vi "Thermometer Readout.vi"() -> ()   [LabVIEW 2023]
uses:
  <vilib>/Utility/file.llb/Read Delimited Spreadsheet (DBL).vi
  MQM Data Transfer All.vi
  Global Variables/Thermometers.vi
panel:
  out "Calibration confirmed":bool
  out "R_H Log Domain":dbl[](array[numeric])
  out "R_H coeffs":dbl[](array[numeric])
  out "Temperatures":cluster{"T_H":dbl, "T_C1":dbl, "T_C2":dbl}
  in  "Stop":bool
  in  "Delay (ms)":dbl=300.0
  in  "T_C2 Lockin":enum16{"LI1", "LI2", "LI3"}(ring)=enum."LI3"
  in  "I_therm":dbl
  in  "T_C1 Lockin":enum16{"LI1", "LI2", "LI3"}(ring)=enum."LI2"
  in  "T_H Lockin":enum16{"LI1", "LI2", "LI3"}(ring)
  out "R_C2 Log Domain":dbl[](array[numeric])
  out "R_C1 Log Domain":dbl[](array[numeric])
  out "R_C2 coeffs":dbl[](array[numeric])
  out "R_C1 coeffs":dbl[](array[numeric])
  in  "R_H domain file":path
  in  "R_C2 domain file":path
  in  "R_C1 domain file":path
  in  "R_C2 coeffs file":path
  in  "R_C1 coeffs file":path
  in  "R_H coeffs file":path
  in  "Confirm Calibration":bool
  in  "Field selection":u16(ring) items=["0.000000"]
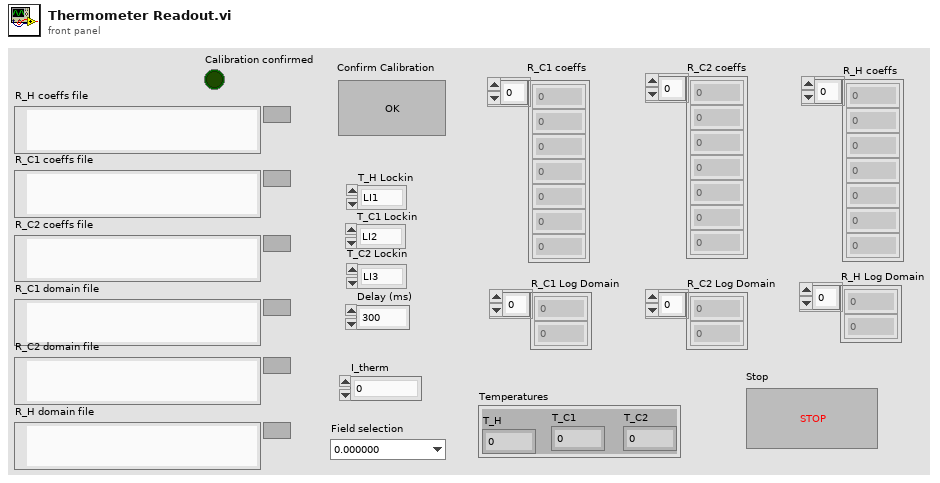
[diagram p1: front panel]
types:
  T1 = cluster{"R_C2 Log Domain":dbl[], "R_C2 coeffs":dbl[], "R_H Log Domain":dbl[], "R_H coeffs":dbl[], "R_C1 Log Domain":dbl[], "R_C1 coeffs":dbl[]}
  T2 = cluster{"T_C2 Lockin":enum16{"LI1", "LI2", "LI3"}, "T_H Lockin":enum16{"LI1", "LI2", "LI3"}, "T_C1 Lockin":enum16{"LI1", "LI2", "LI3"}}
  T3 = typedef "ZI_Frontpanel_All.ctl" = cluster{"Lockin 1 Demod 0":cluster{"R(V)":dbl, "Theta (deg)":dbl, "Timestamp (ms)":u32, "X(V)":dbl, "Y(V)":dbl, "frequency (Hz)":dbl, "output voltage (V)":dbl}, "Lockin 2 Demod 0":cluster{"R(V)":dbl, "Theta (deg)":dbl, "Timestamp (ms)":u32, "X(V)":dbl, "Y(V)":dbl, "frequency (Hz)":dbl, "output voltage (V)":dbl}, "Lockin 3 Demod 0":cluster{"R(V)":dbl, "Theta (deg)":dbl, "Timestamp (ms)":u32, "X(V)":dbl, "Y(V)":dbl, "frequency (Hz)":dbl, "output voltage (V)":dbl}, "Lockin 4 Demod 0":cluster{"R(V)":dbl, "Theta (deg)":dbl, "Timestamp (ms)":u32, "X(V)":dbl, "Y(V)":dbl, "frequency (Hz)":dbl, "output voltage (V)":dbl}, "LI1 active":bool, "LI2 active":bool, "LI3 active":bool, "LI4 active":bool}
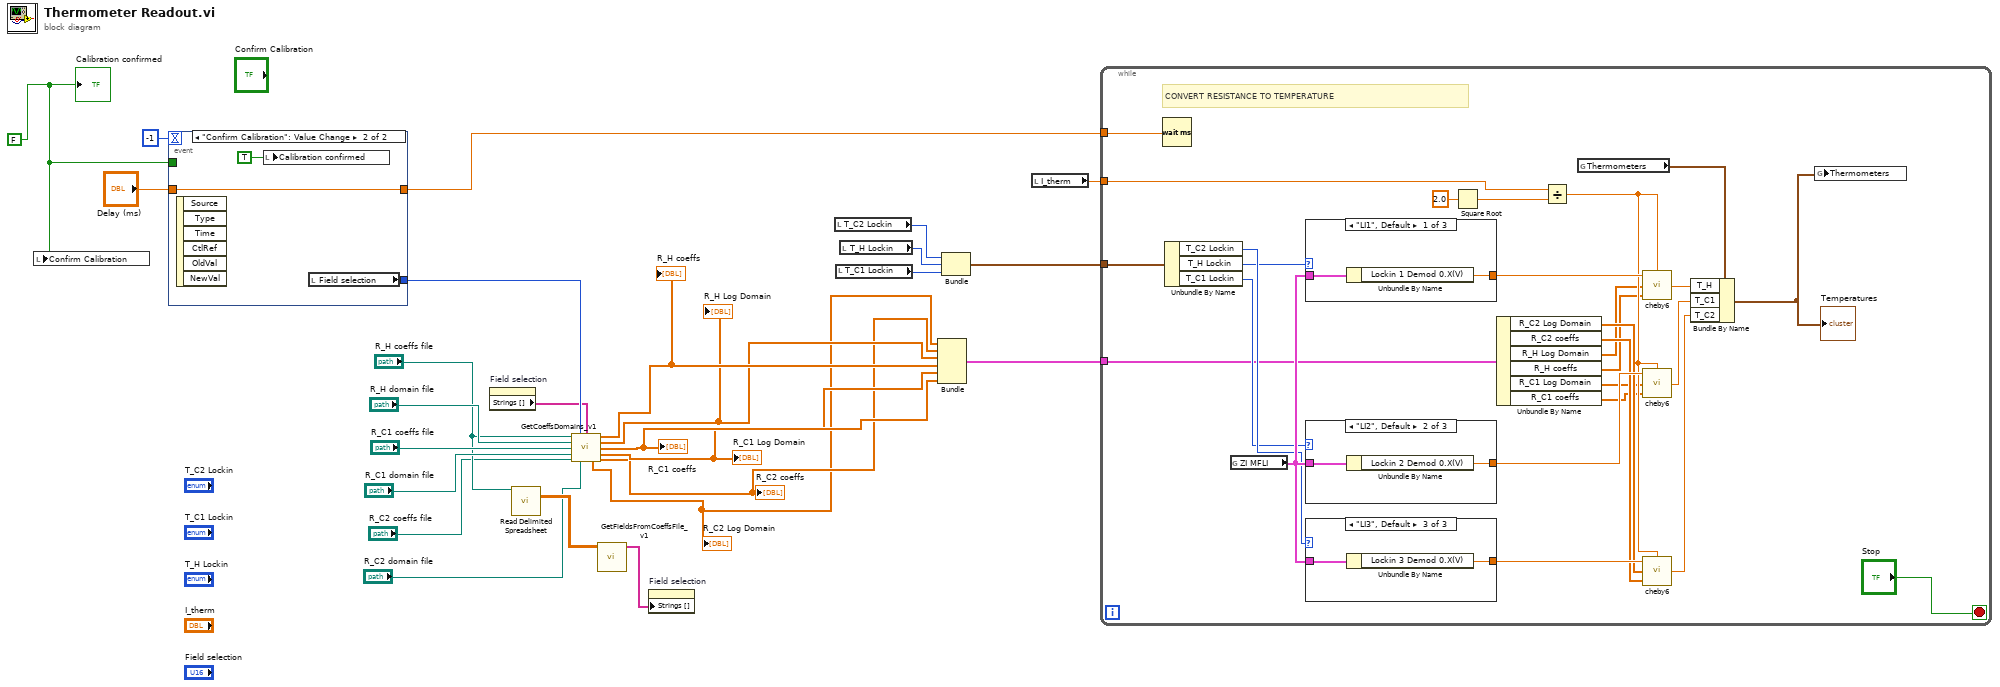
[diagram p0: block diagram]
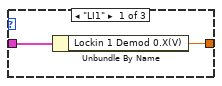
[diagram p2: hidden frame]
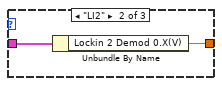
[diagram p3: hidden frame]
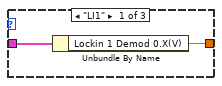
[diagram p4: hidden frame]
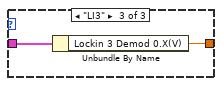
[diagram p5: hidden frame]
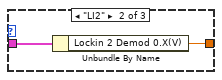
[diagram p6: hidden frame]
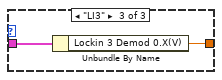
[diagram p7: hidden frame]
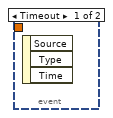
[diagram p8: hidden frame]
diagram:
  w1 = FALSE ("Calibration confirmed")
  n1 = local write "Confirm Calibration"(w1) -> ()
  n2 = event shown="[1] \"Confirm Calibration\": Value Change" {
    selector: _ -> [_ _]
    dyn-events: _ -> [_ _]
    timeout: -1 -> [_ _]
    tunnel: [_ w28] -> w19
    tunnel: "Delay (ms)" -> [_ w27]
    tunnel: [_ w27] -> w8
    tunnel: w1 -> [_ _]
    event Timeout {
      n3 = event-data() -> ()  [unwired: 1 in, 3 out]
    }
    event "Confirm Calibration": Value Change {
      n4 = event-data() -> ()  [unwired: 1 in, 6 out]
      n5 = local write "Calibration confirmed"(TRUE ("Calibration confirmed")) -> ()
      n6 = local read "Field selection"() -> (w28:u16)
    }
  }
  n7 = property on="Field selection" class="Ring (strict)"() -> ("Strings []"=w18:string[])  [unwired: 2 in, 2 out]
  n8 = call-poly <vilib>:"Read Delimited Spreadsheet.vi"("file path (dialog if empty)"="R_H coeffs file") -> ("all rows"=w22:dbl[][])  [unwired: 9 in, 5 out]
  n9 = call "GetCoeffsDomains_v1.vi"("R_H coeffs file"="R_H coeffs file", "Field index"=w19, "Fields"=w18, "R_H domain file"="R_H domain file", "R_C1 coeffs file"="R_C1 coeffs file", "R_C1 domain file"="R_C1 domain file", "R_C2 coeffs file"="R_C2 coeffs file", "R_C2 domain file"="R_C2 domain file") -> ("R_H coeffs"=w7:dbl[], "R_H Log Domain"=w6:dbl[], "R_C1 coeffs"=w5:dbl[], "R_C1 Log Domain"=w4:dbl[], "R_C2 Log Domain"=w2:dbl[], "R_C2 coeffs"=w3:dbl[])  [unwired: 2 in]
  "R_C1 coeffs" <- w5
  "R_C2 coeffs" <- w3
  "R_C1 Log Domain" <- w4
  "R_C2 Log Domain" <- w2
  "R_H coeffs" <- w7
  "R_H Log Domain" <- w6
  n10 = call "GetFieldsFromCoeffsFile_v1.vi"("all rows"=w22) -> ("Array"=w17:string[])  [unwired: 10 in]
  n11 = property on="Field selection" class="Ring (strict)"("Strings []"=w17) -> ()  [unwired: 2 in, 2 out]
  n12 = local read "T_C2 Lockin"() -> (w14:enum16{"LI1", "LI2", "LI3"})
  n13 = local read "T_C1 Lockin"() -> (w12:enum16{"LI1", "LI2", "LI3"})
  n14 = local read "T_H Lockin"() -> (w13:enum16{"LI1", "LI2", "LI3"})
  n15 = Bundle("R_C2 Log Domain"=w2, "R_C2 coeffs"=w3, "R_H Log Domain"=w6, "R_H coeffs"=w7, "R_C1 Log Domain"=w4, "R_C1 coeffs"=w5) -> (w10:T1)  [unwired: 1 in]
  n16 = Bundle("T_C2 Lockin"=w14, "T_H Lockin"=w13, "T_C1 Lockin"=w12) -> (w11:T2)  [unwired: 1 in]
  n17 = local read "I_therm"() -> (w15:dbl)
  n18 = while {
    tunnel: w15 -> [w48]
    tunnel: w11 -> [w42]
    tunnel: w10 -> [w38]
    tunnel: w8 -> [w30]
    stop <- "Stop" stop-if-true
    # "CONVERT RESISTANCE TO TEMPERATURE"
    n19 = Wait (ms)(milliseconds to wait=w30) -> ()  [unwired: 1 out]
    n20 = Unbundle By Name(w42) -> ("T_C2 Lockin"=w41:enum16{"LI1", "LI2", "LI3"}, "T_H Lockin"=w40:enum16{"LI1", "LI2", "LI3"}, "T_C1 Lockin"=w39:enum16{"LI1", "LI2", "LI3"})
    n21 = global read "MQM Data Transfer All.vi" "ZI MFLI"() -> (w49:T3)
    n22 = case shown="\"LI1\", Default" w40 {
      tunnel: w49 -> [w69 w70 w73]
      tunnel: [w68 w71 w72] -> w53
      frame "LI1", Default {
        n23 = Unbundle By Name(w69) -> ("Lockin 1 Demod 0.X(V)"=w68:dbl)
      }
      frame "LI2" {
        n24 = Unbundle By Name(w70) -> ("Lockin 2 Demod 0.X(V)"=w71:dbl)
      }
      frame "LI3" {
        n25 = Unbundle By Name(w73) -> ("Lockin 3 Demod 0.X(V)"=w72:dbl)
      }
    }
    n26 = case shown="\"LI2\", Default" w39 {
      tunnel: w49 -> [w63 w65 w67]
      tunnel: [w62 w64 w66] -> w52
      frame "LI1" {
        n27 = Unbundle By Name(w63) -> ("Lockin 1 Demod 0.X(V)"=w62:dbl)
      }
      frame "LI2", Default {
        n28 = Unbundle By Name(w65) -> ("Lockin 2 Demod 0.X(V)"=w64:dbl)
      }
      frame "LI3" {
        n29 = Unbundle By Name(w67) -> ("Lockin 3 Demod 0.X(V)"=w66:dbl)
      }
    }
    n30 = case shown="\"LI3\", Default" w41 {
      tunnel: w49 -> [w57 w58 w61]
      tunnel: [w56 w59 w60] -> w51
      frame "LI1" {
        n31 = Unbundle By Name(w57) -> ("Lockin 1 Demod 0.X(V)"=w56:dbl)
      }
      frame "LI2" {
        n32 = Unbundle By Name(w58) -> ("Lockin 2 Demod 0.X(V)"=w59:dbl)
      }
      frame "LI3", Default {
        n33 = Unbundle By Name(w61) -> ("Lockin 3 Demod 0.X(V)"=w60:dbl)
      }
    }
    n34 = Square Root(x=2.0) -> (sqrt(x)=w55:dbl)
    n35 = Unbundle By Name(w38) -> ("R_C2 Log Domain"=w37:dbl[], "R_C2 coeffs"=w36:dbl[], "R_H Log Domain"=w35:dbl[], "R_H coeffs"=w34:dbl[], "R_C1 Log Domain"=w33:dbl[], "R_C1 coeffs"=w32:dbl[])
    n36 = Divide(x=w48, y=w55) -> (x/y=w50:dbl)
    n37 = global read "Thermometers.vi" "Thermometers"() -> (w47:cluster{"T_H":dbl, "T_C1":dbl, "T_C2":dbl})
    n38 = call "cheby6.vi"("I"=w50, "Coefs"=w34, "RU/L"=w35, "LIX"=w53) -> ("T"=w46:dbl)
    n39 = call "cheby6.vi"("I"=w50, "Coefs"=w32, "RU/L"=w33, "LIX"=w52) -> ("T"=w44:dbl)
    n40 = call "cheby6.vi"("I"=w50, "Coefs"=w36, "RU/L"=w37, "LIX"=w51) -> ("T"=w45:dbl)
    n41 = Bundle By Name(cluster=w47, "T_H"=w46, "T_C1"=w44, "T_C2"=w45) -> (w43:cluster{"T_H":dbl, "T_C1":dbl, "T_C2":dbl})
    "Temperatures" <- w43
    n42 = global write "Thermometers.vi" "Thermometers"(w43) -> ()
  }
  "Calibration confirmed" <- w1
